vi "and.vi"() -> ()   [LabVIEW 2015]
panel:
  in  "Boolean 3":bool
  in  "Boolean 2":bool
  out "Boolean":bool
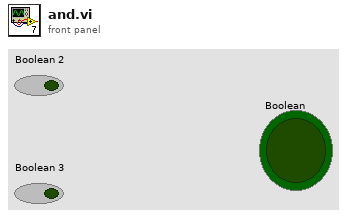
[diagram p1: front panel]
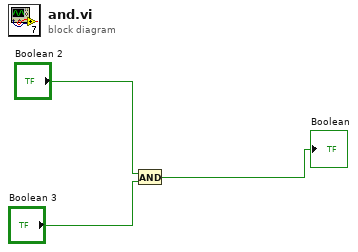
[diagram p0: block diagram]
diagram:
  n1 = And(x="Boolean 2", y="Boolean 3") -> (x .and. y?=→"Boolean":bool)
